vi "Sub_Jacobi_Method.vi"(10 "Max Rotation":i32, 11 "C Matrix":T1) -> (3 "Eigenvalues":dbl[](array[numeric]))   [LabVIEW 2019]
uses:
  <vilib>/Analysis/Matrix/Datatypes/RealMatrix.ctl
  <vilib>/Analysis/Matrix/NI_Matrix.lvlib
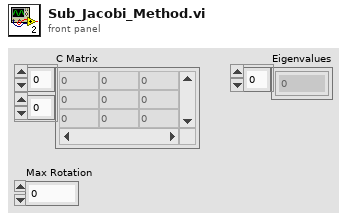
[diagram p1: front panel]
types:
  T1 = typedef "NI_Matrix.lvlib/RealMatrix.ctl" = dbl[][]
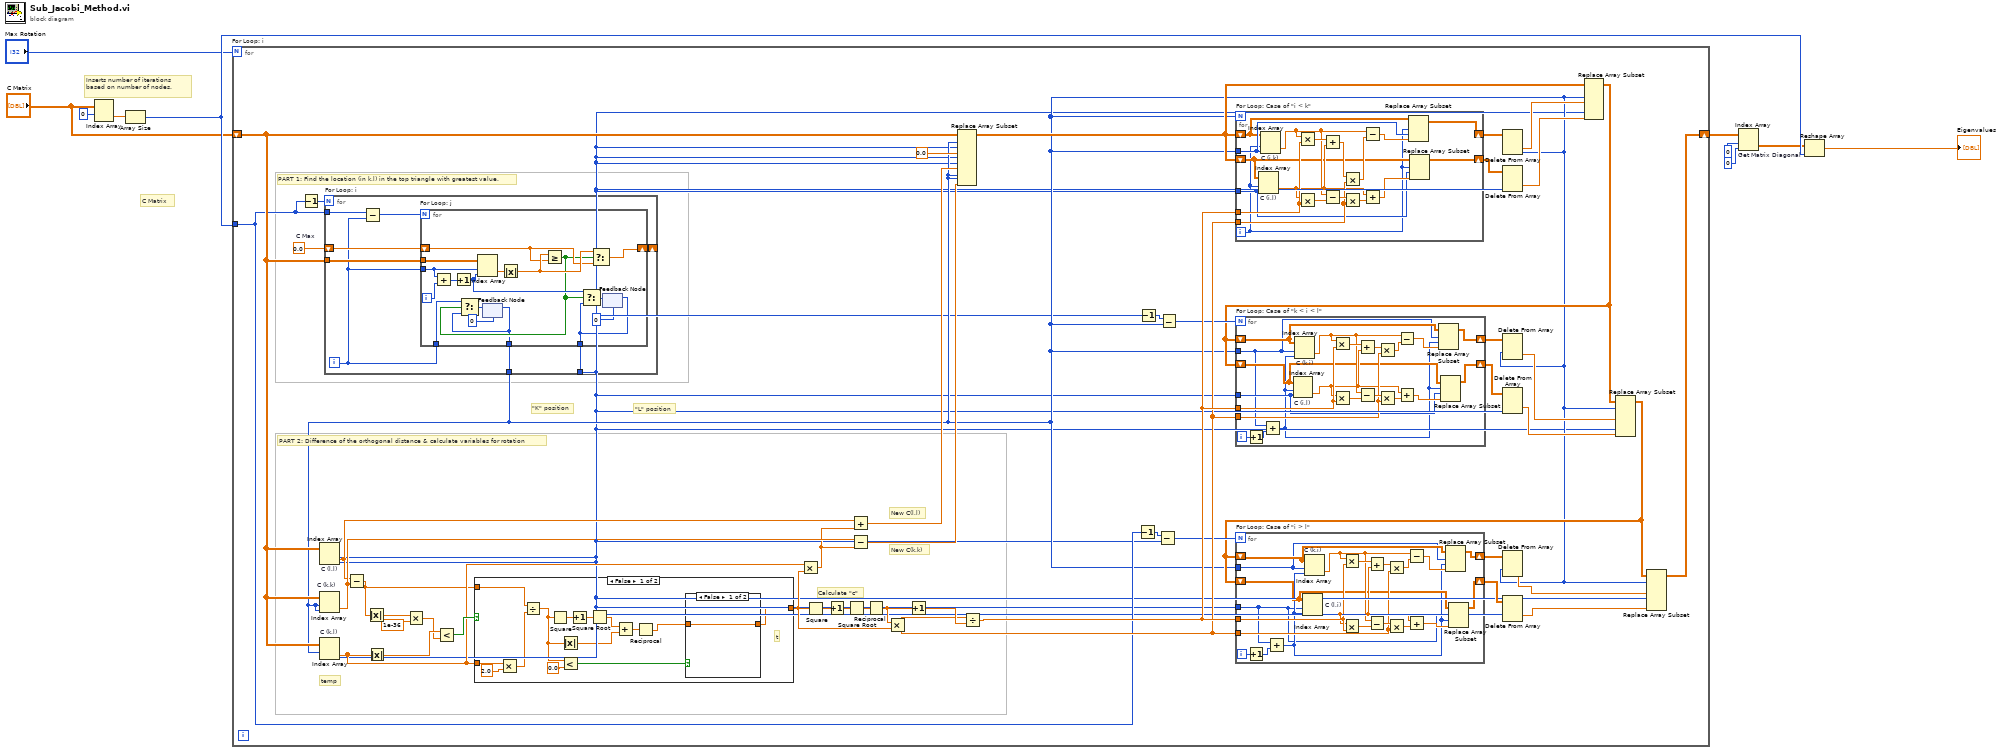
[diagram p0: block diagram]
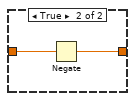
[diagram p2: hidden frame]
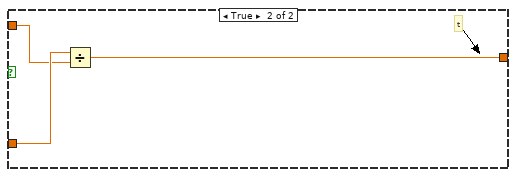
[diagram p3: hidden frame]
diagram:
  # "C Matrix"
  # "Inserts number of iterations\nbased on number of nodes."
  n1 = Index Array(array="C Matrix", index (row)=0) -> (element=w1:dbl[])  [unwired: 1 in]
  n2 = Array Size(array=w1) -> (size(s)=w9:i32)
  n3 = for "For Loop: i" {
    N: "Max Rotation" -> [_]
    tunnel: w9 -> [w13]
    shift-right: [w17] -> w10
    shift-left: "C Matrix" -> [w35]
    w56 = 0.0  # C Max
    # "\"L\" position"
    # "\"K\" position"
    # "PART 2: Difference of the orthogonal distance & calculate variables for rotation"
    # "PART 1: Find the location (in k,l) in the top triangle with greatest value."
    # "New C(l,l)"
    # "New C(k,k)"
    # "temp"
    # "Calculate \"c\""
    n4 = Decrement(x=w13) -> (x-1=w57:i32)
    n5 = for "For Loop: i" {
      N: w57 -> [_]
      tunnel: w35 -> [w146]
      tunnel: w13 -> [w139]
      shift-right: [w144] -> _
      shift-left: w56 -> [w142]
      tunnel: [w143] -> w11
      tunnel: [w141] -> w12
      i -> [w140]
      n6 = Subtract(x=w139, y=w140) -> (x-y=w145:i32)
      n7 = for "For Loop: j" {
        N: w145 -> [_]
        tunnel: w146 -> [w162]
        tunnel: w140 -> [w159]
        shift-right: [w156] -> w144
        shift-left: w142 -> [w157]
        tunnel: [w153] -> w143
        tunnel: [w150] -> w141
        tunnel: w140 -> [w149]
        i -> [w161]
        n8 = Add(x=w159, y=w161) -> (x+y=w160:i32)
        n9 = Increment(x=w160) -> (x+1=w155:i32)
        n10 = Index Array(array=w162, index (row)=w159, index (col)=w155) -> (element=w163:dbl)
        n11 = feedback #1(0) -> (w150:i32)
        n12 = Absolute Value(x=w163) -> (abs(x)=w158:dbl)
        n13 = Greater Or Equal?(x=w158, y=w157) -> (x >= y?=w151:bool)
        n14 = Select(t=w149, s=w151, f=w150) -> (s? t:f=w152:i32)
        n15 = feedback-in #1(w152) -> ()
        n16 = Select(t=w158, s=w151, f=w157) -> (s? t:f=w156:dbl)
        n17 = feedback #2(0) -> (w153:i32)
        n18 = Select(t=w155, s=w151, f=w153) -> (s? t:f=w154:i32)
        n19 = feedback-in #2(w154) -> ()
      }
    }
    n20 = Index Array "C (l,l)"(array=w35, index (row)=w11, index (col)=w11) -> (element=w41:dbl)
    n21 = Index Array "C (k,k)"(array=w35, index (row)=w12, index (col)=w12) -> (element=w45:dbl)
    n22 = Index Array "C (k,l)"(array=w35, index (row)=w12, index (col)=w11) -> (element=w44:dbl)
    n23 = Subtract(x=w41, y=w45) -> (x-y=w36:dbl)
    n24 = Absolute Value(x=w36) -> (abs(x)=w53:dbl)
    n25 = Absolute Value(x=w44) -> (abs(x)=w55:dbl)
    n26 = Multiply(x=w53, y=1e-36 ("x")) -> (x*y=w54:dbl)
    n27 = Less?(x=w55, y=w54) -> (x < y?=w51:bool)
    n28 = case shown="False" w51 {
      tunnel: w44 -> [w132 w138]
      tunnel: w36 -> [w129 w137]
      tunnel: [w119 w136] -> w43
      frame False {
        # "t"
        n29 = Multiply(x=w132, y=2.0) -> (x*y=w130:dbl)
        n30 = Divide(x=w129, y=w130) -> (x/y=w123:dbl)
        n31 = Square(x=w123) -> (x^2=w127:dbl)
        n32 = Absolute Value(x=w123) -> (abs(x)=w128:dbl)
        n33 = Less?(x=w123, y=0.0) -> (x < y?=w121:bool)
        n34 = Increment(x=w127) -> (x+1=w126:dbl)
        n35 = Square Root(x=w126) -> (sqrt(x)=w125:dbl)
        n36 = Add(x=w125, y=w128) -> (x+y=w124:dbl)
        n37 = Reciprocal(x=w124) -> (1/x=w120:dbl)
        n38 = case shown="False" w121 {
          tunnel: w120 -> [w133 w135]
          tunnel: [w133 w134] -> w119
          frame False {
          }
          frame True {
            n39 = Negate(x=w135) -> (-x=w134:dbl)
          }
        }
      }
      frame True {
        # "t"
        n40 = Divide(x=w138, y=w137) -> (x/y=w136:dbl)
      }
    }
    n41 = Multiply(x=w44, y=w43) -> (x*y=w42:dbl)
    n42 = Square(x=w43) -> (x^2=w50:dbl)
    n43 = Increment(x=w50) -> (x+1=w49:dbl)
    n44 = Square Root(x=w49) -> (sqrt(x)=w48:dbl)
    n45 = Add(x=w41, y=w42) -> (x+y=w33:dbl)
    n46 = Subtract(x=w45, y=w42) -> (x-y=w34:dbl)
    n47 = Reciprocal(x=w48) -> (1/x=w47:dbl)
    n48 = Multiply(x=w47, y=w43) -> (x*y=w39:dbl)
    n49 = Increment(x=w47) -> (x+1=w46:dbl)
    n50 = Replace Array Subset(array=w35, new element #1=0.0 ("new element/subarray"), index (row) #1=w12, index (col) #1=w11, new element #2=w33, index (row) #2=w11, index (col) #2=w11, new element #3=w34, index (row) #3=w12, index (col) #3=w12) -> (w28:T1)
    n51 = Divide(x=w39, y=w46) -> (x/y=w40:dbl)
    n52 = Decrement(x=w13) -> (x-1=w14:i32)
    n53 = Decrement(x=w11) -> (x-1=w15:i32)
    n54 = Subtract(x=w14, y=w11) -> (x-y=w38:i32)
    n55 = Subtract(x=w15, y=w12) -> (x-y=w37:i32)
    n56 = for "For Loop: Case of \"i < k\"" {
      N: w12 -> [_]
      tunnel: w40 -> [w115]
      tunnel: w39 -> [w112]
      tunnel: w12 -> [w107]
      tunnel: w11 -> [w102]
      shift-right: [w105] -> w32
      shift-left: w28 -> [w106]
      shift-right: [w101] -> w31
      shift-left: w28 -> [w104]
      i -> [w100]
      n57 = Index Array "C (i,l)"(array=w104, index (row)=w100, index (col)=w102) -> (element=w109:dbl)
      n58 = Index Array "C (i,k)"(array=w106, index (row)=w100, index (col)=w107) -> (element=w110:dbl)
      n59 = Multiply(x=w110, y=w115) -> (x*y=w118:dbl)
      n60 = Multiply(x=w109, y=w115) -> (x*y=w114:dbl)
      n61 = Add(x=w118, y=w109) -> (x+y=w117:dbl)
      n62 = Subtract(x=w110, y=w114) -> (x-y=w113:dbl)
      n63 = Multiply(x=w117, y=w112) -> (x*y=w116:dbl)
      n64 = Multiply(x=w113, y=w112) -> (x*y=w111:dbl)
      n65 = Subtract(x=w110, y=w116) -> (x-y=w108:dbl)
      n66 = Add(x=w109, y=w111) -> (x+y=w103:dbl)
      n67 = Replace Array Subset(array=w106, new element=w108, index (row)=w100, index (col)=w107) -> (w105:T1)
      n68 = Replace Array Subset(array=w104, new element=w103, index (row)=w100, index (col)=w102) -> (w101:T1)
    }
    n69 = Delete From Array(array=w32, index (col)=w12) -> (deleted portion=w29:dbl[])  [unwired: 2 in, 1 out]
    n70 = Delete From Array(array=w31, index (col)=w11) -> (deleted portion=w30:dbl[])  [unwired: 2 in, 1 out]
    n71 = Replace Array Subset(array=w28, new element #1=w29, index (col) #1=w12, new element #2=w30, index (col) #2=w11) -> (w25:T1)  [unwired: 2 in]
    n72 = for "For Loop: Case of \"k < i < l\"" {
      N: w37 -> [_]
      tunnel: w40 -> [w96]
      tunnel: w39 -> [w93]
      tunnel: w11 -> [w83]
      tunnel: w12 -> [w81]
      shift-right: [w87] -> w24
      shift-left: w25 -> [w89]
      shift-right: [w86] -> w23
      shift-left: w25 -> [w85]
      i -> [w80]
      n73 = Increment(x=w80) -> (x+1=w79:i32)
      n74 = Add(x=w81, y=w79) -> (x+y=w82:i32)
      n75 = Index Array "C (i,l)"(array=w85, index (row)=w82, index (col)=w83) -> (element=w90:dbl)
      n76 = Index Array "C (k,i)"(array=w89, index (row)=w81, index (col)=w82) -> (element=w91:dbl)
      n77 = Multiply(x=w91, y=w96) -> (x*y=w99:dbl)
      n78 = Multiply(x=w90, y=w96) -> (x*y=w95:dbl)
      n79 = Add(x=w99, y=w90) -> (x+y=w98:dbl)
      n80 = Subtract(x=w91, y=w95) -> (x-y=w94:dbl)
      n81 = Multiply(x=w98, y=w93) -> (x*y=w97:dbl)
      n82 = Multiply(x=w94, y=w93) -> (x*y=w92:dbl)
      n83 = Subtract(x=w91, y=w97) -> (x-y=w88:dbl)
      n84 = Add(x=w90, y=w92) -> (x+y=w84:dbl)
      n85 = Replace Array Subset(array=w89, new element=w88, index (row)=w81, index (col)=w82) -> (w87:T1)
      n86 = Replace Array Subset(array=w85, new element=w84, index (row)=w82, index (col)=w83) -> (w86:T1)
    }
    n87 = Delete From Array(array=w24, index (row)=w12) -> (deleted portion=w26:dbl[])  [unwired: 2 in, 1 out]
    n88 = Delete From Array(array=w23, index (col)=w11) -> (deleted portion=w27:dbl[])  [unwired: 2 in, 1 out]
    n89 = Replace Array Subset(array=w25, new element #1=w26, index (row) #1=w12, new element #2=w27, index (col) #2=w11) -> (w22:T1)  [unwired: 2 in]
    n90 = for "For Loop: Case of \"i > l\"" {
      N: w38 -> [_]
      tunnel: w40 -> [w75]
      tunnel: w39 -> [w72]
      tunnel: w12 -> [w66]
      tunnel: w11 -> [w60]
      shift-right: [w65] -> w21
      shift-left: w22 -> [w68]
      shift-right: [w63] -> w20
      shift-left: w22 -> [w64]
      i -> [w59]
      n91 = Increment(x=w59) -> (x+1=w58:i32)
      n92 = Add(x=w60, y=w58) -> (x+y=w61:i32)
      n93 = Index Array "C (l,i)"(array=w64, index (row)=w60, index (col)=w61) -> (element=w69:dbl)
      n94 = Index Array "C (k,i)"(array=w68, index (row)=w66, index (col)=w61) -> (element=w70:dbl)
      n95 = Multiply(x=w70, y=w75) -> (x*y=w78:dbl)
      n96 = Multiply(x=w69, y=w75) -> (x*y=w74:dbl)
      n97 = Add(x=w78, y=w69) -> (x+y=w77:dbl)
      n98 = Subtract(x=w70, y=w74) -> (x-y=w73:dbl)
      n99 = Multiply(x=w77, y=w72) -> (x*y=w76:dbl)
      n100 = Multiply(x=w73, y=w72) -> (x*y=w71:dbl)
      n101 = Subtract(x=w70, y=w76) -> (x-y=w67:dbl)
      n102 = Add(x=w69, y=w71) -> (x+y=w62:dbl)
      n103 = Replace Array Subset(array=w68, new element=w67, index (row)=w66, index (col)=w61) -> (w65:T1)
      n104 = Replace Array Subset(array=w64, new element=w62, index (row)=w60, index (col)=w61) -> (w63:T1)
    }
    n105 = Delete From Array(array=w21, index (row)=w12) -> (deleted portion=w19:dbl[])  [unwired: 2 in, 1 out]
    n106 = Delete From Array(array=w20, index (row)=w11) -> (deleted portion=w18:dbl[])  [unwired: 2 in, 1 out]
    n107 = Replace Array Subset(array=w22, new element #1=w19, index (row) #1=w12, new element #2=w18, index (row) #2=w11) -> (w17:T1)  [unwired: 2 in]
  }
  n108 = Index Array "Get Matrix Diagonal"(array=w10, index (row)=0, index (col)=0) -> (element=w5:T1)
  n109 = Reshape Array(w5, w9) -> (→"Eigenvalues":dbl[])
